vi "READ File.vi"(0 "reference in":refnum<class "Nastran PCH.lvclass">, 5 "error in (no error)":errorcluster, 7 "F07 File Path - READ":path) -> (14 "reference out":refnum<class "Nastran PCH.lvclass">, 19 "error out":errorcluster)   [LabVIEW 2020, in "Nastran PCH.lvclass"]
uses:
  Nastran PCH.lvclass
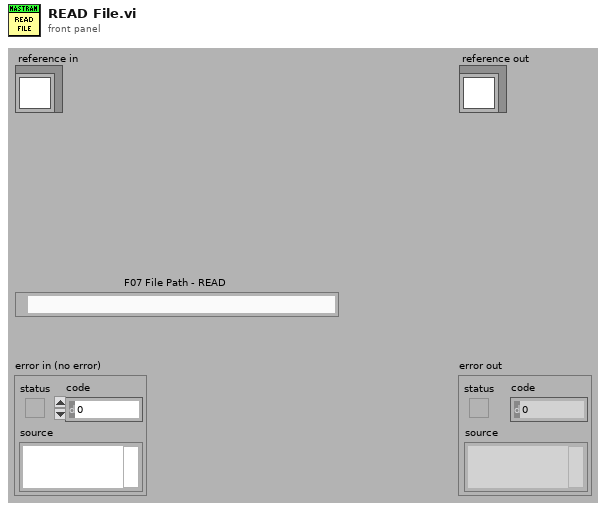
[diagram p1: front panel]
types:
  T1 = typedef "Nastran PCH.lvclass/ObjectAttributesRef.ctl" = refnum<data-value>
  T2 = cluster{"Header Start":i32, "DATA Start":i32, "Header Length":i32, "DATA Length":i32}[]
  T3 = cluster{"Title":string, "Sub Title":string, "Point ID":i32, "Subcase ID":i32, "Name":string, "Unit Type":enum16{"displacement", "velocity", "acceleration"}, "Unit":string, "Storage Type":enum16{"Sort1", "Sort2"}, "Abscissa":dbl[], "X":cdb[], "Y":cdb[], "Z":cdb[], "u":cdb[], "v":cdb[], "w":cdb[]}[]
  T4 = typedef "Nastran PCH.lvclass/ObjectAttributes.ctl" = cluster{"FRF":cluster{"Title":string, "Sub Title":string, "Point ID":i32, "Subcase ID":i32, "Name":string, "Unit Type":enum16{"displacement", "velocity", "acceleration"}, "Unit":string, "Storage Type":enum16{"Sort1", "Sort2"}, "Abscissa":dbl[], "X":cdb[], "Y":cdb[], "Z":cdb[], "u":cdb[], "v":cdb[], "w":cdb[]}[]}
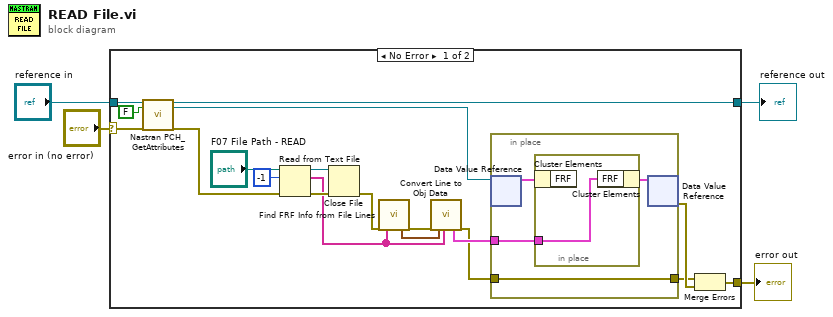
[diagram p0: block diagram]
diagram:
  n1 = case shown="No Error" "error in (no error)" {
    selector: "error in (no error)" -> [w18 w30]
    tunnel: [w23 w30] -> w3
    tunnel: [w17 w29] -> w1
    tunnel: "reference in" -> [w20 w29]
    frame No Error {
      n2 = call "Nastran PCH_GetAttributes.vi"("reference in"=w20, "return data? (T)"=FALSE, "error in (no error)"=w18) -> ("reference out"=w17:refnum<class "Nastran PCH.lvclass">, "attributes ref"=w16:T1, "error out"=w11:errorcluster)  [unwired: 13 in, 1 out]
      n3 = Read from Text File(file (use dialog)="F07 File Path - READ", count=-1, error in=w11) -> (refnum out=w14:refnum<file>, text=w7:string[], error out=w13:errorcluster)  [unwired: 1 in, 1 out]
      n4 = Close File(refnum=w14, error in=w13) -> (error out=w10:errorcluster)  [unwired: 1 out]
      n5 = call "Find FRF Info from File Lines.vi"("error in (no error)"=w10, "Line text"=w7) -> ("Channel Lines info"=w8:T2, "error out"=w9:errorcluster)  [unwired: 16 in]
      n6 = call "Convert Line to Obj Data.vi"("error in (no error)"=w9, "Channel Lines info"=w8, "Line text"=w7) -> ("FRF"=w6:T3, "error out"=w5:errorcluster)  [unwired: 15 in]
      n7 = in-place {
        in-place-border: w5 -> [w25]
        in-place-border: [w25] -> w21
        in-place-border: w6 -> [w24]
        n8 = in-place-dvr #1(w16) -> (w26:T4)  [unwired: 1 out]
        n9 = in-place {
          in-place-border: w24 -> [w28]
          n10 = in-place-cluster #2(w26) -> ()  [unwired: 1 out]
          n11 = in-place-cluster #2("FRF"=w28) -> (w27:T4)
        }
        n12 = in-place-dvr #1(w27) -> (w22:errorcluster)  [unwired: 1 out]
      }
      n13 = Merge Errors(w21, w22) -> (w23:errorcluster)
    }
    frame Error {
    }
  }
  "error out" <- w3
  "reference out" <- w1
